vi "FPGA Main.vi"() -> ()   [LabVIEW 2018]
doc: "This VI contains a control loop running in parallel with an RT watchdog loop.\n- The 'Control Loop' performs control calculations on two input channels in parallel, and outputs the results to two output channels.\n- The 'RT Watchdog' Loop checks for a periodic 'pet' from the RT Main VI to ensure communications between RT and the FPGA are maintained."
uses:
  controls/FPGA State.ctl
  controls/Control Configuration.ctl
  controls/Raw Values.ctl
  <vilib>/rvi/Emulation/niFpgaGetClockAttributes.vi
  <vilib>/rvi/Emulation/niFpgaSctlEmulationGetInTimedLoop.vi
  <vilib>/rvi/Emulation/niFpgaEmulationReportErrorSimple.vi
  <vilib>/rvi/Emulation/niFpgaProcessEmulError.vi
  <vilib>/rvi/eio/common/nirviEmuTemplateMethod_errors.vi
  <vilib>/rvi/Emulation/niFpgaCriticalErrorInLSC.vi
  <vilib>/eio/EIONode/EIONode.xnode
panel:
  in  "Channel 1 Setpoint":fxp<+/-,16,5>
  in  "Channel 0 Setpoint":fxp<+/-,16,5>
  out "Watchdog Timed Out?":bool=TRUE
  in  "Enable Watchdog":bool
  in  "Pet Watchdog":bool
  in  "Watchdog Timeout Period (ticks)":u64=40000000 format="%.0p"
  out "Time Since Last Pet":u64
  out "Output Values":T1
  out "Input Values":T1
  in  "Channel 1 Configuration":T2={"PID Gains"={"proportional gain (Kc)"=0.0, "integral gain (Kc*Ts/Ti)"=0.0, "derivative gain (Kc*Td/Ts)"=0.0}, "Output Range"={"output high"=10.0, "output low"=-10.0}}
  in  "Channel 0 Configuration":T2={"PID Gains"={"proportional gain (Kc)"=0.0, "integral gain (Kc*Ts/Ti)"=0.0, "derivative gain (Kc*Td/Ts)"=0.0}, "Output Range"={"output high"=10.0, "output low"=-10.0}}
  in  "New State":T3=enum."Control (PID)"
  out "Actual Loop Period (ticks)":u32
  out "Current FPGA State":T3=enum."Control (PID)"
  in  "Change State":bool
  out "Input Error":bool
  out "Output Error":bool
  in  "Control Period (ticks)":u32
  # "General Settings"
  # "Monitoring Values"
  # "Watchdog Settings"
  # "Control Settings"
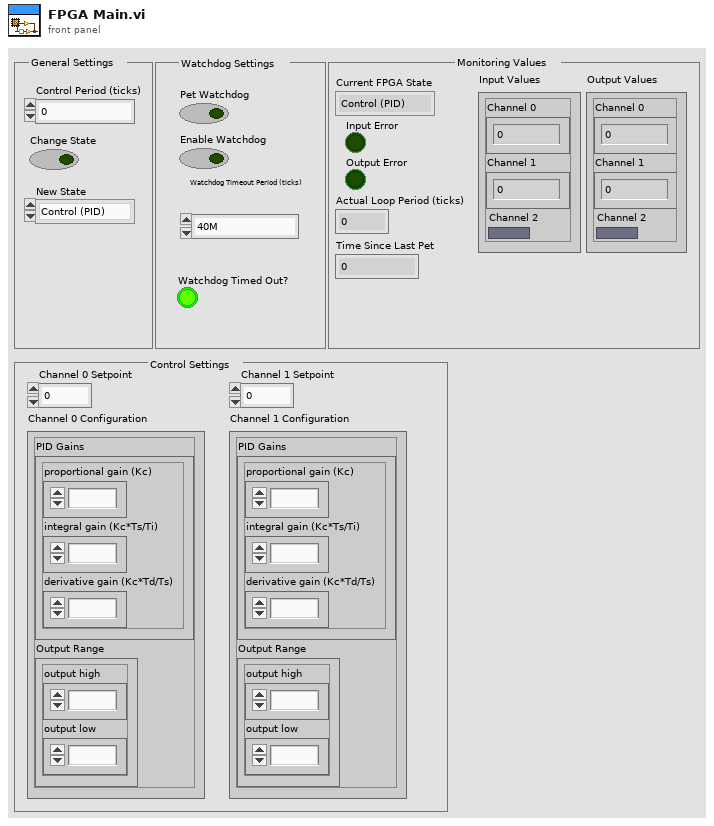
[diagram p1: front panel]
types:
  T1 = typedef "Raw Values.ctl" = cluster{"Channel 0":fxp<+/-,20,5>, "Channel 1":fxp<+/-,20,5>, "Channel 2":bool}
  T2 = typedef "Control Configuration.ctl" = cluster{"PID Gains":cluster{"proportional gain (Kc)":fxp<+/-,16,8>, "integral gain (Kc*Ts/Ti)":fxp<+/-,16,8>, "derivative gain (Kc*Td/Ts)":fxp<+/-,16,8>}, "Output Range":cluster{"output high":fxp<+/-,16,5>, "output low":fxp<+/-,16,5>}}
  T3 = typedef "FPGA State.ctl" = enum16{"Safe State", "Control (PID)"}
  T4 = cluster{"proportional gain (Kc)":fxp<+/-,16,8>, "integral gain (Kc*Ts/Ti)":fxp<+/-,16,8>, "derivative gain (Kc*Td/Ts)":fxp<+/-,16,8>}
  T5 = cluster{"output high":fxp<+/-,16,5>, "output low":fxp<+/-,16,5>}
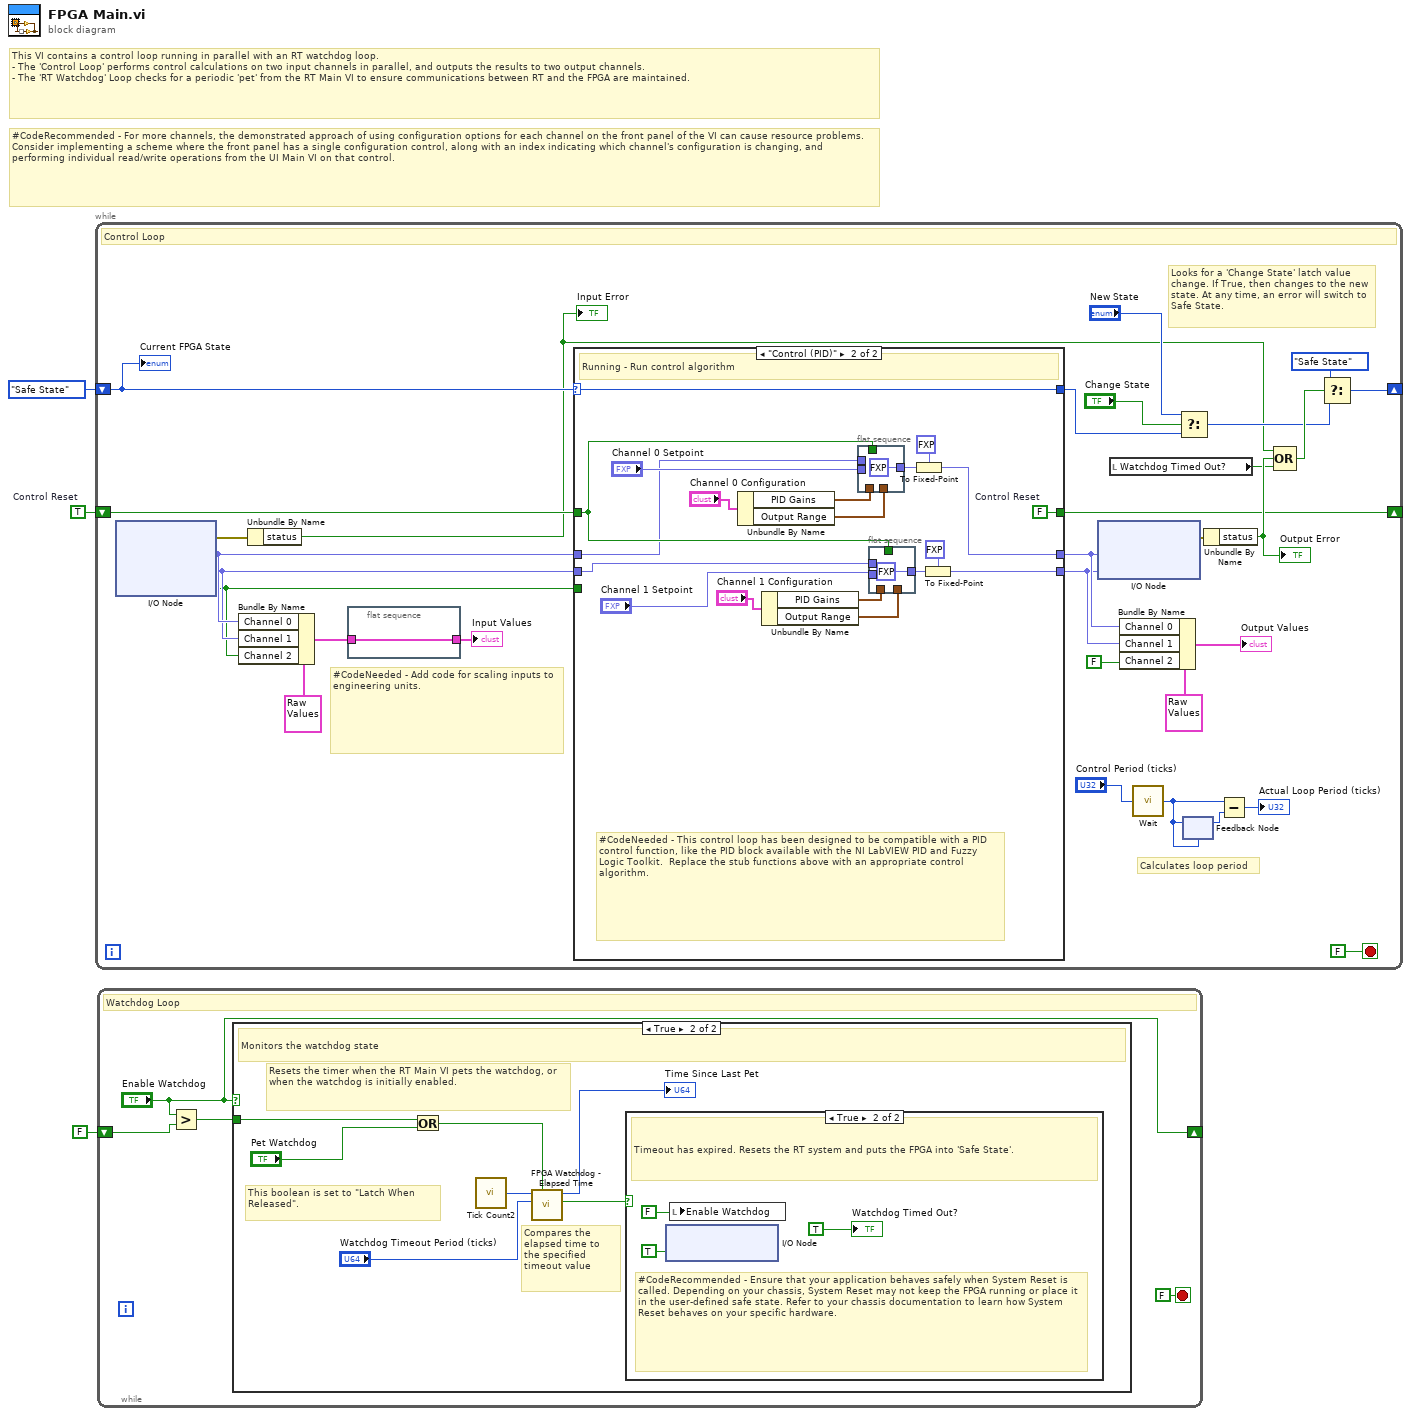
[diagram p0: block diagram]
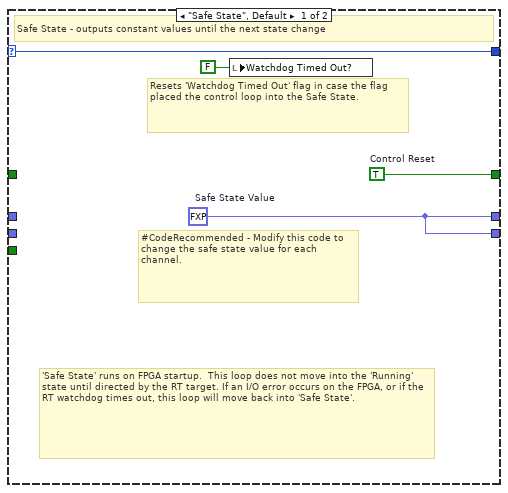
[diagram p4: hidden frame]
diagram:
  w2 = TRUE  # Control Reset
  # "#CodeRecommended - For more channels, the demonstrated approach of using configuration options for each channel on the front panel of the VI can cause resource problems.  Consider implementing a scheme where the front panel has a single configuration control, along with an index indicating which channel's configuration is changing, and performing individual read/write operations from the UI Main VI on that control."
  # "This VI contains a control loop running in parallel with an RT watchdog loop.\n- The 'Control Loop' performs control calculations on two input channels in parallel, and outputs the results to two output channels.\n- The 'RT Watchdog' Loop checks for a periodic 'pet' from the RT Main VI to ensure communications between RT and the FPGA are maintained."
  n1 = while {
    shift-right: [w29] -> _
    shift-left: FPGA_State."Safe State" ("FPGA State") -> [w20]
    shift-right: [w26] -> _
    shift-left: w2 -> [w25]
    stop <- FALSE stop-if-true
    # "Looks for a 'Change State' latch value change. If True, then changes to the new state. At any time, an error will switch to Safe State."
    # "#CodeNeeded - Add code for scaling inputs to engineering units."
    # "Calculates loop period"
    # "Control Loop"
    n2 = xnode "I/O Node"() -> ("error out"=w33:errorcluster, "Mod1/AI0"=w18:fxp<+/-,16,5>, "Mod4/TC0"=w17:fxp<+/-,24,-2>, "Mod3/DI0"=w16:bool)  [unwired: 4 in, 3 out]
    n3 = Bundle By Name(cluster=T1 {"Channel 0"=0.0, "Channel 1"=0.0, "Channel 2"=FALSE} ("Raw Values"), "Channel 0"=w18, "Channel 1"=w17, "Channel 2"=w16) -> (w5:T1)
    n4 = Unbundle By Name(w33) -> ("status"=w19:bool)
    "Input Error" <- w19
    n5 = flat-sequence {
      tunnel: [w35] -> w4
      tunnel: w5 -> [w35]
      frame #0 {
      }
    }
    n6 = case shown="\"Control (PID)\"" w20 {
      selector: w20 -> [w38 w55]
      tunnel: w18 -> [_ w42]
      tunnel: [w37 w57] -> w15
      tunnel: [w38 w55] -> w24
      tunnel: [w39 w56] -> w26
      tunnel: w25 -> [_ w44]
      tunnel: w17 -> [_ w43]
      tunnel: w16 -> [_ _]
      tunnel: [w37 w51] -> w14
      frame "Safe State", Default {
        w37 = fxp<+/-,20,5> 0.0  # Safe State Value
        w39 = TRUE  # Control Reset
        # "'Safe State' runs on FPGA startup.  This loop does not move into the 'Running' state until directed by the RT target. If an I/O error occurs on the FPGA, or if the RT watchdog times out, this loop will move back into 'Safe State'."
        # "Resets 'Watchdog Timed Out' flag in case the flag placed the control loop into the Safe State."
        # "#CodeRecommended - Modify this code to change the safe state value for each channel."
        # "Safe State - outputs constant values until the next state change"
        n7 = local write "Watchdog Timed Out?"(FALSE ("Watchdog Timed Out?")) -> ()
      }
      frame "Control (PID)" {
        w56 = FALSE  # Control Reset
        # "#CodeNeeded - This control loop has been designed to be compatible with a PID control function, like the PID block available with the NI LabVIEW PID and Fuzzy Logic Toolkit.  Replace the stub functions above with an appropriate control algorithm."
        # "Running - Run control algorithm"
        n8 = Unbundle By Name("Channel 0 Configuration") -> ("PID Gains"=w47:T4, "Output Range"=w46:T5)
        n9 = Unbundle By Name("Channel 1 Configuration") -> ("PID Gains"=w50:T4, "Output Range"=w49:T5)
        n10 = flat-sequence {
          tunnel: w47 -> [_]
          tunnel: w46 -> [_]
          tunnel: "Channel 0 Setpoint" -> [_]
          tunnel: w44 -> [_]
          tunnel: w42 -> [_]
          tunnel: [fxp<+/-,16,5> 0.0 ("output")] -> w40
          frame #0 {
          }
        }
        n11 = flat-sequence {
          tunnel: w50 -> [_]
          tunnel: w49 -> [_]
          tunnel: "Channel 1 Setpoint" -> [_]
          tunnel: w44 -> [_]
          tunnel: w43 -> [_]
          tunnel: [fxp<+/-,16,5> 0.0 ("output")] -> w41
          frame #0 {
          }
        }
        n12 = To Fixed-Point(fixed-point type=fxp<+/-,20,5> 0.0 ("Off Value"), number=w40) -> (fixed-point=w57:fxp<+/-,20,5>)
        n13 = To Fixed-Point(fixed-point type=fxp<+/-,20,5> 0.0 ("Off Value"), number=w41) -> (fixed-point=w51:fxp<+/-,20,5>)
      }
    }
    n14 = xnode "I/O Node"("Mod2/AO0"=w15, "Mod2/AO1"=w14) -> ("error out"=w32:errorcluster)  [unwired: 3 in, 2 out]
    n15 = local read "Watchdog Timed Out?"() -> (w12:bool)
    n16 = Bundle By Name(cluster=T1 {"Channel 0"=0.0, "Channel 1"=0.0, "Channel 2"=FALSE} ("Raw Values"), "Channel 0"=w15, "Channel 1"=w14, "Channel 2"=FALSE) -> (→"Output Values":T1)
    n17 = call "Wait"("Count(Ticks)"="Control Period (ticks)") -> ("Tick Count(Ticks)"=w11:u32)
    n18 = Select(t="New State", s="Change State", f=w24) -> (s? t:f=w21:T3)
    n19 = feedback-in #1(w11) -> ()
    n20 = feedback #1(w11) -> (w10:u32)
    n21 = Unbundle By Name(w32) -> ("status"=w31:bool)
    "Output Error" <- w31
    n22 = Subtract(x=w11, y=w10) -> (x-y=→"Actual Loop Period (ticks)":u32)
    n23 = Compound Arithmetic op=OR(w19, w31, w12) -> (w28:bool)
    n24 = Select(t=FPGA_State."Safe State" ("FPGA State"), s=w28, f=w21) -> (s? t:f=w29:T3)
    "Current FPGA State" <- w20
    "Input Values" <- w4
  }
  n25 = while "RT Watchdog Loop" {
    shift-right: ["Enable Watchdog"] -> _
    shift-left: FALSE ("Enable RT Watchdog") -> [w64]
    stop <- FALSE stop-if-true
    # "Watchdog Loop"
    n26 = Greater?(x="Enable Watchdog", y=w64) -> (0:w61:bool)
    n27 = case shown="True" "Enable Watchdog" {
      tunnel: w61 -> [_ w67]
      frame False {
        # "This loop has to be explicitly enabled from the RT Main VI.  This reduces the possibility of an endless restart cycle."
      }
      frame True {
        # "This boolean is set to \"Latch When Released\"."
        # "Compares the elapsed time to the specified timeout value"
        # "Resets the timer when the RT Main VI pets the watchdog, or when the watchdog is initially enabled."
        # "Monitors the watchdog state"
        n28 = Or(x=w67, y="Pet Watchdog") -> (x .or. y?=w66:bool)
        n29 = call "Tick Count2"() -> ("Tick Count(Ticks)"=w70:u32)
        n30 = call "FPGA Watchdog - Elapsed Time.vi"("Reset"=w66, "Timeout Period"="Watchdog Timeout Period (ticks)", "Current Time"=w70) -> ("Timeout"=w65:bool, "Elapsed Time"=→"Time Since Last Pet":u64)  [unwired: 7 in]
        n31 = case shown="True" w65 {
          frame False {
            # "Timeout has not expired."
          }
          frame True {
            # "#CodeRecommended - Ensure that your application behaves safely when System Reset is called. Depending on your chassis, System Reset may not keep the FPGA running or place it in the user-defined safe state. Refer to your chassis documentation to learn how System Reset behaves on your specific hardware."
            # "Timeout has expired. Resets the RT system and puts the FPGA into 'Safe State'."
            n32 = xnode "I/O Node"("System Reset"=TRUE ("RT Reset on Watchdog Failure?")) -> ()  [unwired: 1 in, 1 out]
            n33 = local write "Enable Watchdog"(FALSE ("Enable RT Watchdog")) -> ()
            "Watchdog Timed Out?" <- TRUE ("Watchdog Timed Out?")
          }
        }
      }
    }
  }
